vi "send_multiple_queue.vi"(8 "error in (no error)":errorcluster, 9 "Processing":refnum<queue>, 10 "RFID":refnum<queue>, 11 "info":cluster{"File path":T1, "Cfg ":T2} {"Cfg"."Offset_rueda WS 2" format="%.27g"; "Cfg"."Offset_rueda WS 1" format="%.27g"; "Cfg"."Frecuencia de muestreo y módulo CRIO" items=["51.200 kS/s (NI 9234)"=1, "25.600 kS/s (NI 9234)"=2, "17.067 kS/s (NI 9234)"=3, "12.800 kS/s (NI 9234)"=4, "10.240 kS/s (NI 9234)"=5, "8.533 kS/s (NI 9234)"=6, "7.314 kS/s (NI 9234)"=7, "6.400 kS/s (NI 9234)"=8, "5.689 kS/s (NI 9234)"=9, "5.120 kS/s (NI 9234)"=10, "4.654 kS/s (NI 9234)"=11, "4.267 kS/s (NI 9234)"=12, "3.938 kS/s (NI 9234)"=13, "3.657 kS/s (NI 9234)"=14, "3.413 kS/s (NI 9234)"=15, "3.200 kS/s (NI 9234)"=16, "3.012 kS/s (NI 9234)"=17, "2.845 kS/s (NI 9234)"=18, "2.695 kS/s (NI 9234)"=19, "2.560 kS/s (NI 9234)"=20, "2.438 kS/s (NI 9234)"=21, "2.328 kS/s (NI 9234)"=22, "2.226 kS/s (NI 9234)"=23, "2.133 kS/s (NI 9234)"=24, "2.048 kS/s (NI 9234)"=25, "1.969 kS/s (NI 9234)"=26, "1.896 kS/s (NI 9234)"=27, "1.829 kS/s (NI 9234)"=28, "1.765 kS/s (NI 9234)"=29, "1.707 kS/s (NI 9234)"=30, "1.652 kS/s (NI 9234)"=31]}) -> (0 "error out":errorcluster)   [LabVIEW 2015]
uses:
  controls/File paths.ctl
  controls/Cfg_parameters.ctl
  <vilib>/LabVIEW Targets/FPGA/cRIO/shared/nicrio_ModuleControls/nicrio_cRIO-9234_DataRatesRing2.ctl
  Message Queue/Message Cluster.ctl
  Message Queue/Enqueue Message (Single).vi
  Message Queue/Message Queue.lvlib
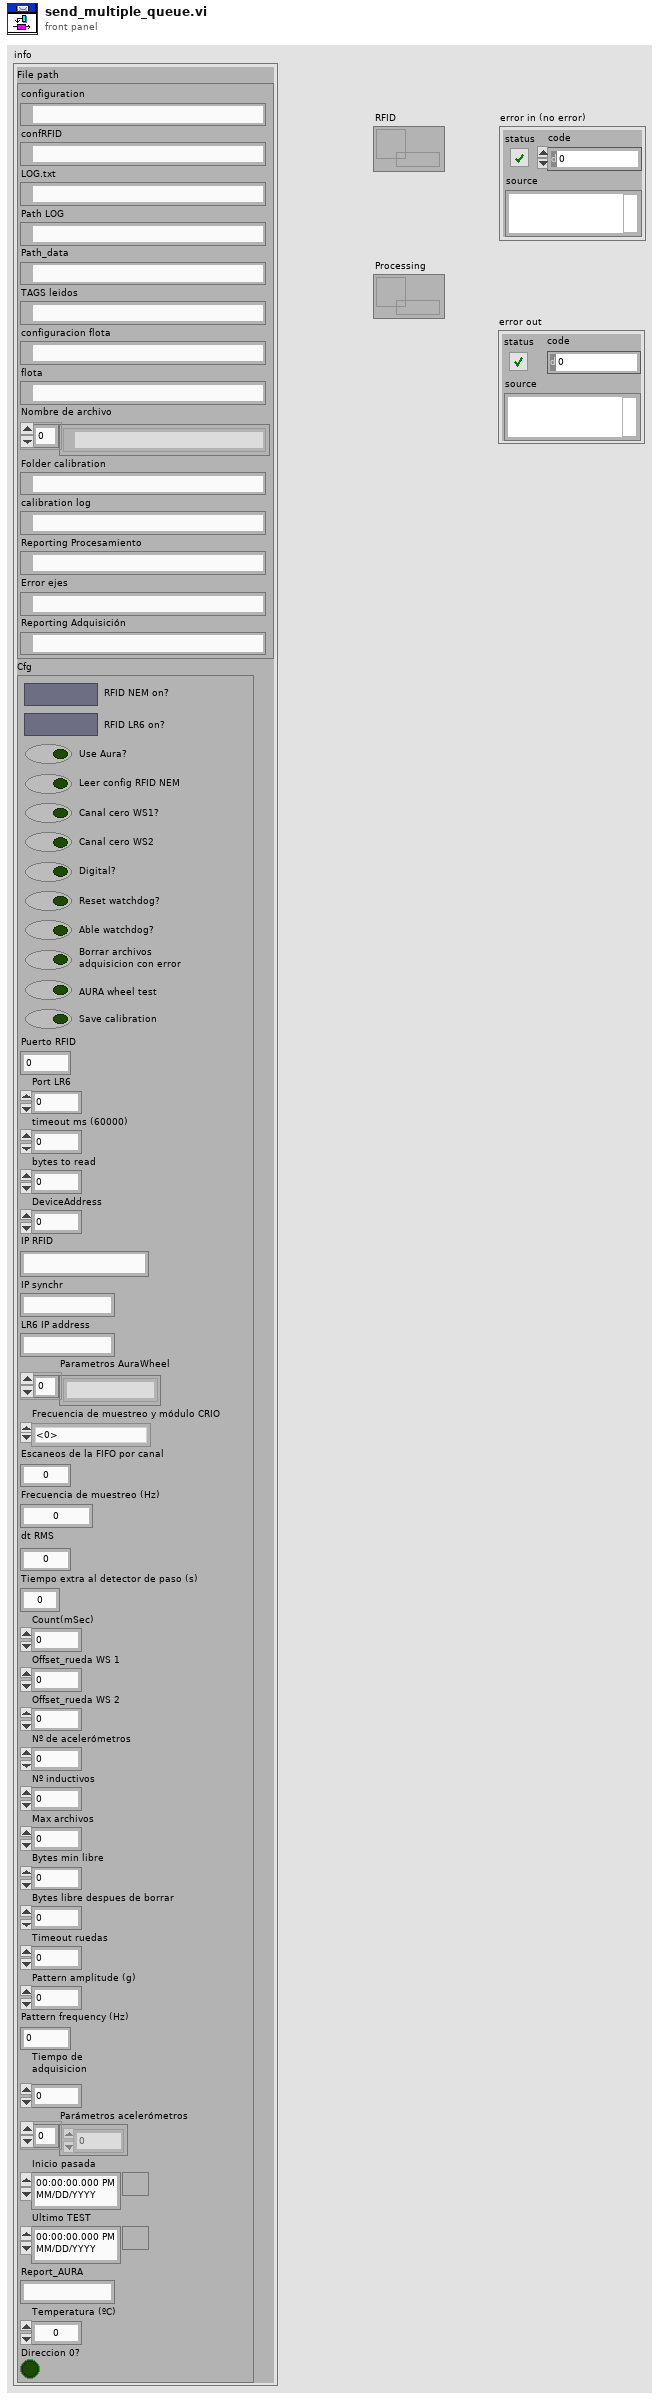
[diagram p1: front panel]
types:
  T1 = typedef "File paths.ctl" = cluster{"configuration":path, "confRFID":path, "LOG.txt":path, "Path LOG":path, "Path_data":path, "TAGS leidos":path, "configuracion flota":path, "flota":path, "Nombre de archivo":path[], "Folder calibration":path, "calibration log":path, "Reporting Procesamiento":path, "Error ejes":path, "Reporting Adquisición":path}
  T2 = typedef "Cfg_parameters.ctl" = cluster{"RFID NEM on?":bool, "RFID LR6 on?":bool, "Use Aura?":bool, "Leer config RFID NEM":bool, "Canal cero WS1?":bool, "Canal cero WS2 ":bool, "Digital?":bool, "Reset watchdog?":bool, "Able watchdog?":bool, "Borrar archivos\nadquisicion con error":bool, "AURA wheel test":bool, "Save calibration":bool, "Puerto RFID":u16, "Port LR6":u16, "timeout ms (60000)":i32, "bytes to read":i32, "DeviceAddress":u8, "IP RFID":string, "IP synchr":string, "LR6 IP address":string, "Parametros AuraWheel":string[], "Frecuencia de muestreo y módulo CRIO":T3, "Escaneos de la FIFO por canal":u32, "Frecuencia de muestreo (Hz)":dbl, "dt RMS":dbl, "Tiempo extra al detector de paso (s)":dbl, "Count(mSec)":u32, "Offset_rueda WS 1":fxp<+/-,24,-4>, "Offset_rueda WS 2":fxp<+/-,24,-4>, "Nº de acelerómetros":i32, "Nº inductivos":i32, "Max archivos":u32, "Bytes min libre":u32, "Bytes libre despues de borrar":u32, "Timeout ruedas":dbl, "Pattern amplitude (g)":dbl, "Pattern frequency (Hz)":dbl, "Tiempo de adquisicion\n":dbl, "Parámetros acelerómetros":dbl[], "Inicio pasada":timestamp, "Ultimo TEST":timestamp, "Report_AURA":string, "Temperatura (ºC)":dbl, "Direccion 0?":bool}
  T3 = typedef "nicrio_cRIO-9234_DataRatesRing2.ctl" = u8
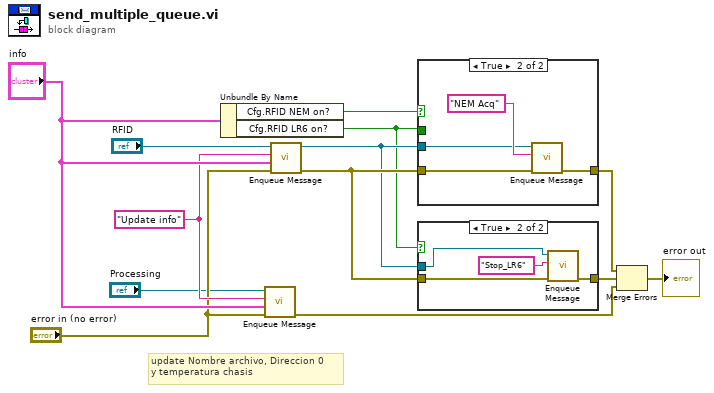
[diagram p0: block diagram]
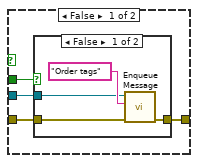
[diagram p3: hidden frame]
diagram:
  w10 = "Update info" ("Message")
  # "update Nombre archivo, Direccion 0\ny temperatura chasis"
  n1 = Unbundle By Name("info") -> ("Cfg.RFID NEM on?"=w6:bool, "Cfg.RFID LR6 on?"=w1:bool)
  n2 = call-poly "Enqueue Message.vi"("error in (no error)"="error in (no error)", "Message Data"="info", "Message"=w10, "Message Queue"="Processing") -> ("error out"=w7:errorcluster)  [unwired: 6 in, 1 out]
  n3 = call-poly "Enqueue Message.vi"("error in (no error)"="error in (no error)", "Message Data"="info", "Message"=w10, "Message Queue"="RFID") -> ("error out"=w5:errorcluster, "dup Message Queue"=w4:refnum<queue>)  [unwired: 6 in]
  n4 = case shown="True" w6 {
    tunnel: [w16 w26] -> w12
    tunnel: w5 -> [w17 w25]
    tunnel: w4 -> [w14 w23]
    tunnel: w1 -> [w15 _]
    frame False {
      n5 = case shown="False" w15 {
        tunnel: [w19 w22] -> w16
        tunnel: w17 -> [w20 w22]
        tunnel: w14 -> [w18 _]
        frame False {
          n6 = call-poly "Enqueue Message.vi"("error in (no error)"=w20, "Message"="Order tags", "Message Queue"=w18) -> ("error out"=w19:errorcluster)  [unwired: 7 in, 1 out]
        }
        frame True {
        }
      }
    }
    frame True {
      n7 = call-poly "Enqueue Message.vi"("error in (no error)"=w25, "Message"="NEM Acq", "Message Queue"=w23) -> ("error out"=w26:errorcluster)  [unwired: 7 in, 1 out]
    }
  }
  n8 = case shown="True" w1 {
    tunnel: [w27 w31] -> w8
    tunnel: w5 -> [w27 w30]
    tunnel: w4 -> [_ w28]
    frame False {
    }
    frame True {
      n9 = call-poly "Enqueue Message.vi"("error in (no error)"=w30, "Message"="Stop_LR6", "Message Queue"=w28) -> ("error out"=w31:errorcluster)  [unwired: 7 in, 1 out]
    }
  }
  n10 = Merge Errors(w12, w8, w7) -> (→"error out":errorcluster)
